vi "MainControl.vi"(11 "Marlin COM port":refnum<visa-resource-name>) -> (3 "Marin Serial Response":string)   [LabVIEW 2020]
uses:
  <vilib>/Instr/_visa.llb/VISA Configure Serial Port (Instr).vi
panel:
  in  "Add Command":string
  in  "Poll Temps":bool
  out "Sent Command\n( HEX )":string
  out "Sent Command\n( ASCII )":string
  out "Iteration No":i32
  out "Commands\nFIFO Buffer":string[](array[string])
  out "Bed\n( °C )":dbl(slide) scale=0.0..50.0
  out "PP Extdr.\n( °C )":dbl(slide) scale=0.0..50.0
  in  "stop":bool
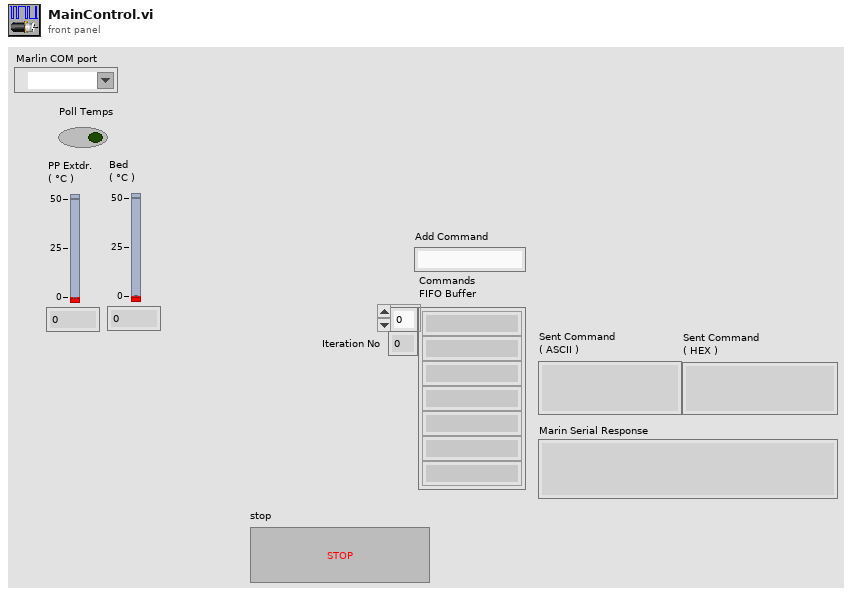
[diagram p1: front panel]
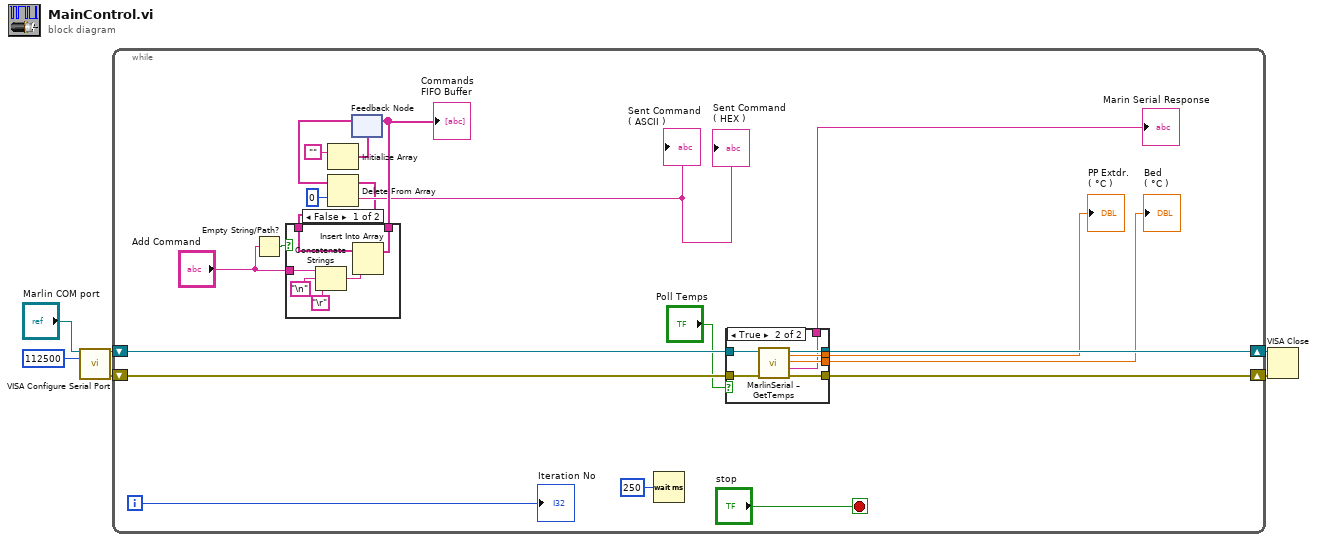
[diagram p0: block diagram]
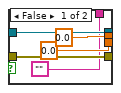
[diagram p3: hidden frame]
diagram:
  n1 = call-poly "VISA Configure Serial Port"("VISA resource name"="Marlin COM port", "baud rate (9600)"=u32 112500) -> ("VISA resource name out"=w3:refnum<visa-resource-name>, "error out"=w5:errorcluster)  [unwired: 12 in]
  n2 = while {
    shift-right: [w26] -> w6
    shift-left: w5 -> [w25]
    shift-right: [w24] -> w4
    shift-left: w3 -> [w23]
    i -> [w13]
    stop <- "stop" stop-if-true
    n3 = Empty String/Path?(string/path="Add Command") -> (empty?=w16:bool)
    n4 = Initialize Array("") -> (w14:string[])  [unwired: 1 in]
    n5 = feedback #1(w14) -> (w11:string[])
    n6 = Delete From Array(array=w11, index=0) -> (deleted portion=→"Sent Command\n( ASCII )" →"Sent Command\n( HEX )":string, array with subset deleted=w8:string[])  [unwired: 1 in]
    n7 = case shown="False" w16 {
      tunnel: "Add Command" -> [w28 _]
      tunnel: [w31 w33] -> w12
      tunnel: w8 -> [w32 w33]
      frame False {
        n8 = Concatenate Strings(w28, "\n", "\r") -> (w27:string)
        n9 = Insert Into Array(array=w32, new element=w27) -> (w31:string[])  [unwired: 1 in]
      }
      frame True {
      }
    }
    "Commands\nFIFO Buffer" <- w12
    n10 = feedback-in #1(w12) -> ()
    n11 = Wait (ms)(milliseconds to wait=u32 250) -> ()  [unwired: 1 out]
    n12 = case shown="True" "Poll Temps" {
      tunnel: [w37 w45] -> w26
      tunnel: w25 -> [w37 w44]
      tunnel: [w38 w43] -> w24
      tunnel: w23 -> [w38 w42]
      tunnel: [0.0 ("Grabbed float 2") w41] -> w20
      tunnel: [0.0 ("Grabbed float") w40] -> w19
      tunnel: ["" ("read buffer") w39] -> w18
      frame False {
      }
      frame True {
        n13 = call "MarlinSerial – GetTemps.vi"("error in (no error)"=w44, "VISA Refnum in"=w42) -> ("error out"=w45:errorcluster, "Grabbed float 2"=w41:dbl, "read buffer"=w39:string, "VISA Refnum out"=w43:refnum<visa-resource-name>, "Grabbed float"=w40:dbl)  [unwired: 5 in]
      }
    }
    "Marin Serial Response" <- w18
    "Bed\n( °C )" <- w19
    "PP Extdr.\n( °C )" <- w20
    "Iteration No" <- w13
  }
  n14 = VISA Close(VISA resource name=w4, error in (no error)=w6) -> ()  [unwired: 1 out]
